vi "REPORT_OKNOK_recolor_columns.vi"(6 "Recolor? (T)":bool=TRUE, 8 "error_in":errorcluster, 10 "records":string[][](array[string]), 11 "listbox_ref":refnum<vi>) -> (0 "error_out":errorcluster)   [LabVIEW 2019]
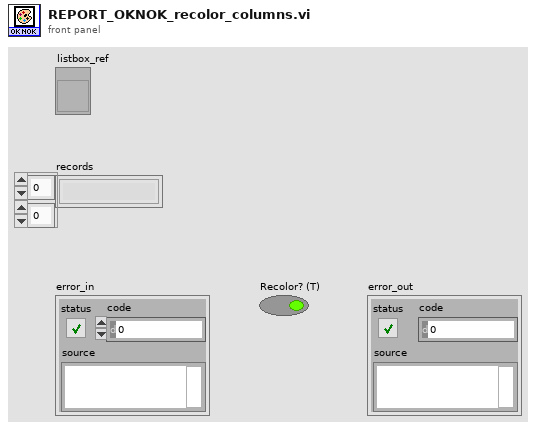
[diagram p1: front panel]
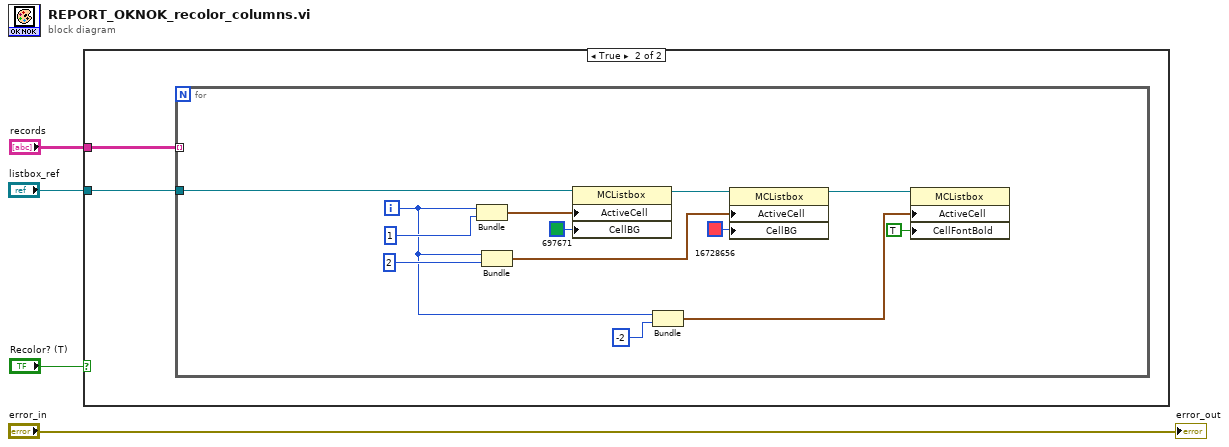
[diagram p0: block diagram]
diagram:
  n1 = case shown="True" "Recolor? (T)" {
    tunnel: "records" -> [_ w5]
    tunnel: "listbox_ref" -> [_ w6]
    frame False {
    }
    frame True {
      n2 = for {
        tunnel: w6 -> [w19]
        tunnel: w5 -> [_] mode=indexing
        i -> [w7]
        n3 = Bundle(w7, 1) -> (w17:cluster{i32, i32})  [unwired: 1 in]
        n4 = Bundle(w7, 2) -> (w15:cluster{i32, i32})  [unwired: 1 in]
        n5 = property on="Property Node" class="MCListbox"(reference=w19, "ActiveCell"=w17, "CellBG"=u32 697671) -> (reference out=w16:refnum<vi>)  [unwired: 1 in, 1 out]
        n6 = Bundle(w7, -2) -> (w11:cluster{i32, i32})  [unwired: 1 in]
        n7 = property on="Property Node" class="MCListbox"(reference=w16, "ActiveCell"=w15, "CellBG"=u32 16728656) -> (reference out=w9:refnum<vi>)  [unwired: 1 in, 1 out]
        n8 = property on="Property Node" class="MCListbox"(reference=w9, "ActiveCell"=w11, "CellFontBold"=TRUE ("Active Cell:Cell Font:Bold")) -> ()  [unwired: 1 in, 2 out]
      }
    }
  }
  "error_out" <- "error_in"
